vi "Add Result Channels.vi"(8 "error in (no error)":errorcluster, 9 "Selected Source Waveforms items":T1[](array[typedef]) format="%.0x", 10 "Selected Waveform Result Section items":T1[](array[typedef]) format="%.0x", 11 "RunningAverageCalculation in":refnum<class "RunningAverageCalculation.lvclass">) -> (0 "error out":errorcluster, 3 "RunningAverageCalculation out":refnum<class "RunningAverageCalculation.lvclass">)   [LabVIEW 2015, in "RunningAverageCalculation.lvclass"]
uses:
  Waveform-Processing-Custom-Device Configuration.llb/RunningAverageCalculation.lvclass
  Waveform-Processing-Custom-Device Configuration.llb/Custom Device Item Ref.ctl
  Waveform-Processing-Custom-Device Configuration.llb/WaveformCalculation.lvclass/WaveformCalculation.ctl
  Waveform-Processing-Custom-Device Configuration.llb/Custom Device Channel.ctl
  Waveform-Processing-Custom-Device Configuration.llb/Custom Device Channel Type.ctl
  Waveform-Processing-Custom-Device Configuration.llb/WaveformCalculation.lvclass
  Waveform-Processing-Custom-Device Configuration.llb/Custom Device API.lvlib
  Waveform-Processing-Custom-Device Configuration.llb/Waveform-Processing-Custom-Device System Explorer.lvlib
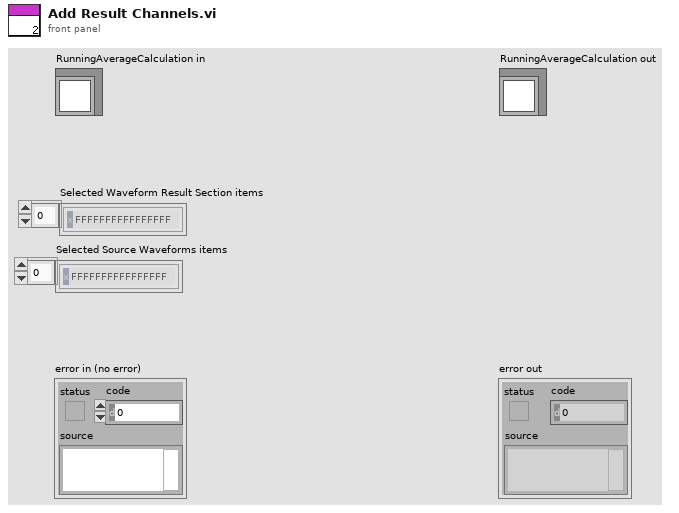
[diagram p1: front panel]
types:
  T1 = typedef "Custom Device API.lvlib/Custom Device Item Ref.ctl" = u64
  T2 = typedef "Custom Device API.lvlib/Custom Device Channel.ctl" = cluster{"Type":T3, "Units":string, "Default Value":dbl, "Faultable":bool, "Scalable":bool}
  T3 = typedef "Custom Device API.lvlib/Custom Device Channel Type.ctl" = enum16{"Input", "Output"}
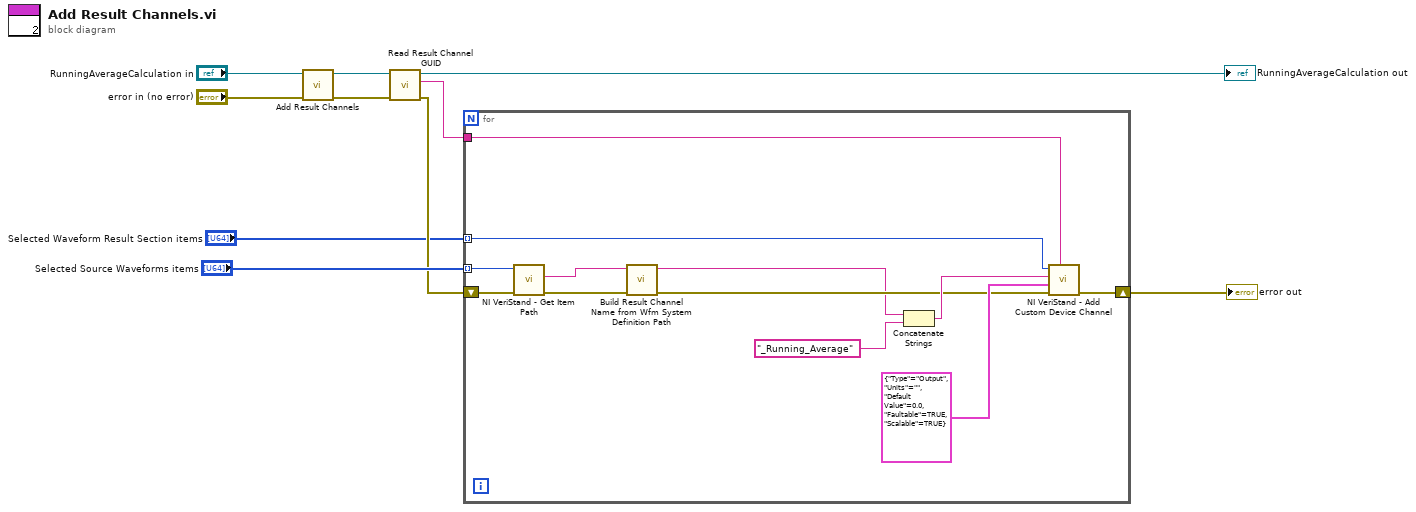
[diagram p0: block diagram]
diagram:
  n1 = call-parent "Add Result Channels.vi"("error in (no error)"="error in (no error)", "WaveformCalculation in"="RunningAverageCalculation in") -> ("error out"=w3:errorcluster, "WaveformCalculation out"=w6:refnum<class "RunningAverageCalculation.lvclass">)  [unwired: 8 in]
  n2 = call "Read Result Channel GUID.vi"("error in (no error)"=w3, "WaveformCalculation in"=w6) -> ("error out"=w9:errorcluster, "Result Channel GUID"=w8:string, "WaveformCalculation out"=→"RunningAverageCalculation out":refnum<class "RunningAverageCalculation.lvclass">)  [unwired: 7 in]
  n3 = for {
    tunnel: "Selected Source Waveforms items" -> [w17] mode=indexing
    shift-right: [w19] -> w1
    shift-left: w9 -> [w18]
    tunnel: w8 -> [w11]
    tunnel: "Selected Waveform Result Section items" -> [w12] mode=indexing
    n4 = call "NI VeriStand - Get Item Path.vi"("error in (no error)"=w18, "Item Ref in"=w17) -> ("error out"=w15:errorcluster, "Path"=w16:string)  [unwired: 6 in, 2 out]
    n5 = call "Build Result Channel Name from Wfm System Definition Path.vi"("error in (no error)"=w15, "Channel Path"=w16) -> ("error out"=w14:errorcluster, "delimited string"=w13:string)  [unwired: 8 in]
    n6 = Concatenate Strings(w13, "_Running_Average" ("string")) -> (w21:string)
    n7 = call "NI VeriStand - Add Custom Device Channel.vi"("GUID (Default Channel)"=w11, "error in (no error)"=w14, "Channel"=T2 {"Type"=enum."Output", "Units"="", "Default Value"=0.0, "Faultable"=TRUE, "Scalable"=TRUE}, "Channel Name"=w21, "Parent Ref in"=w12) -> ("error out"=w19:errorcluster)  [unwired: 3 in, 3 out]
  }
  "error out" <- w1
